vi "Read Individual Data.vi"   [LabVIEW 2020, in "eec 6700.lvlib"]
doc: "Reads the test data individually from the instrument during the test progress."
uses:
  <instrlib>/eec 6700/eec 6700.lvlib
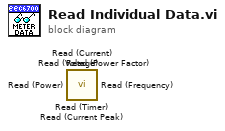
[diagram p0: block diagram]
diagram:
  n1 = call <instrlib>:"Read (Timer).vi"() -> ()  [unwired: 13 in, 3 out]
  n2 = call <instrlib>:"Read (Power Factor).vi"() -> ()  [unwired: 13 in, 3 out]
  n3 = call <instrlib>:"Read (Power).vi"() -> ()  [unwired: 13 in, 3 out]
  n4 = call <instrlib>:"Read (Frequency).vi"() -> ()  [unwired: 13 in, 3 out]
  n5 = call <instrlib>:"Read (Current Peak).vi"() -> ()  [unwired: 13 in, 3 out]
  n6 = call <instrlib>:"Read (Current).vi"() -> ()  [unwired: 13 in, 3 out]
  n7 = call <instrlib>:"Read (Voltage).vi"() -> ()  [unwired: 13 in, 3 out]
